vi "Write SysMsg.vi"(8 "error in (no error)":errorcluster, 10 "SysMsg":string[](array[string]), 11 "xData in":refnum<class "xData.lvclass">) -> (0 "error out":errorcluster, 3 "xData out":refnum<class "xData.lvclass">)   [LabVIEW 2014, in "xData.lvclass"]
uses:
  xData.lvclass
  xData.lvclass/xData.ctl
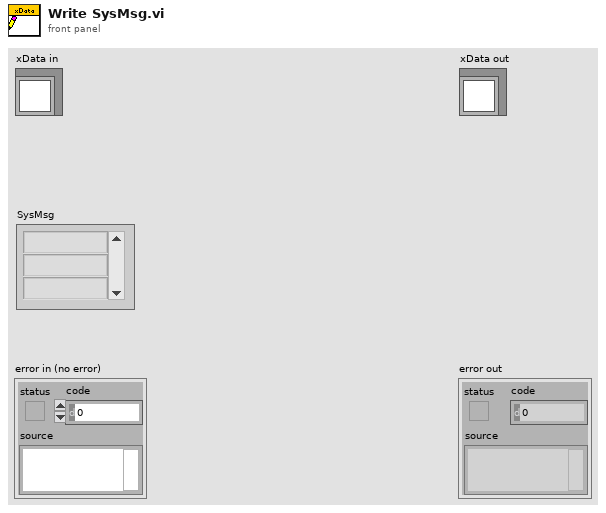
[diagram p1: front panel]
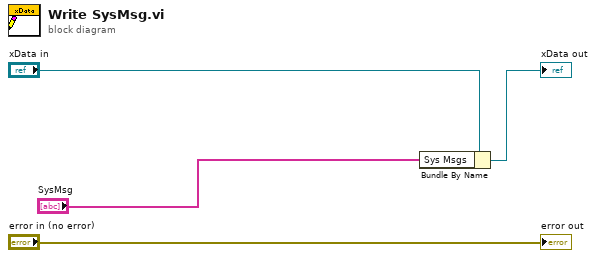
[diagram p0: block diagram]
diagram:
  n1 = Bundle By Name(cluster="xData in", "Sys Msgs"="SysMsg") -> (→"xData out":refnum<class "xData.lvclass">)
  "error out" <- "error in (no error)"
